vi "风速测量.vi"() -> ()   [LabVIEW 2014]
panel:
  in  "DAQmx物理通道":tag
  out "添加的数组":u32[](array[numeric])
  out "Error Out":errorcluster caption="错误输出"
  in  "字符串":string
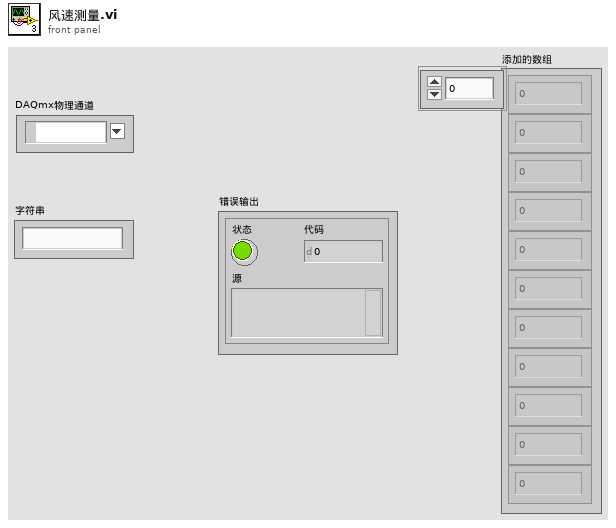
[diagram p1: front panel]
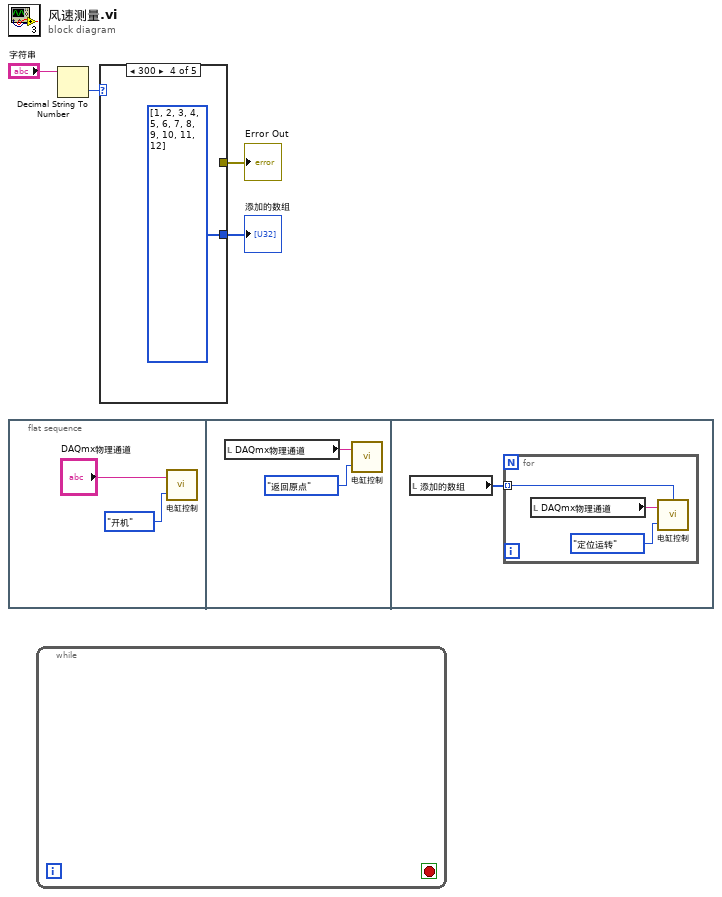
[diagram p0: block diagram]
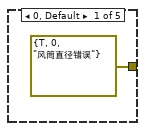
[diagram p2: hidden frame]
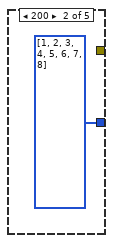
[diagram p3: hidden frame]
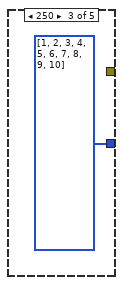
[diagram p4: hidden frame]
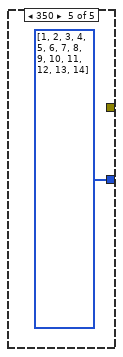
[diagram p5: hidden frame]
diagram:
  n1 = flat-sequence {
    frame #0 {
      n2 = call "电缸控制.vi"("枚举"=enum16{"开机", "返回原点", "定位运转", "报警复位"}."开机", "输出设备"="DAQmx物理通道") -> ()  [unwired: 1 in, 1 out]
    }
    frame #1 {
      n3 = local read "DAQmx物理通道"() -> (w8:tag)
      n4 = call "电缸控制.vi"("枚举"=enum16{"开机", "返回原点", "定位运转", "报警复位"}."返回原点", "输出设备"=w8) -> ()  [unwired: 1 in, 1 out]
    }
    frame #2 {
      n5 = local read "添加的数组"() -> (w9:u32[])
      n6 = for {
        tunnel: w9 -> [w11] mode=indexing
        n7 = local read "DAQmx物理通道"() -> (w12:tag)
        n8 = call "电缸控制.vi"("步序号"=w11, "枚举"=enum16{"开机", "返回原点", "定位运转", "报警复位"}."定位运转", "输出设备"=w12) -> ()  [unwired: 1 out]
      }
    }
  }
  n9 = while {
    stop <- _ stop-if-true
  }
  n10 = Decimal String To Number(string="字符串") -> (number=w3:i32)  [unwired: 2 in, 1 out]
  n11 = case shown="300" w3 {
    tunnel: [errorcluster {"status"=TRUE, "code"=0, "source"="风筒直径错误"} ("Error Out") _ _ _ _] -> w1
    tunnel: [_ i32[] [1, 2, 3, 4, 5, 6, 7, 8] i32[] [1, 2, 3, 4, 5, 6, 7, 8, 9, 10] u32[] [1, 2, 3, 4, 5, 6, 7, 8, 9, 10, 11, 12] i32[] [1, 2, 3, 4, 5, 6, 7, 8, 9, 10, 11, 12, 13, 14]] -> w2
    frame 0, Default {
    }
    frame 200 {
    }
    frame 250 {
    }
    frame 300 {
    }
    frame 350 {
    }
  }
  "Error Out" <- w1
  "添加的数组" <- w2
